vi "Write bestY.vi"(8 "error in (no error)":errorcluster, 10 "bestY":dbl, 11 "Utilities in":refnum<class "Utilities.lvclass">) -> (0 "error out":errorcluster, 3 "Utilities out":refnum<class "Utilities.lvclass">)   [LabVIEW 2023, in "Utilities.lvclass"]
uses:
  Utilities.lvclass
  Utilities.lvclass/Utilities.ctl
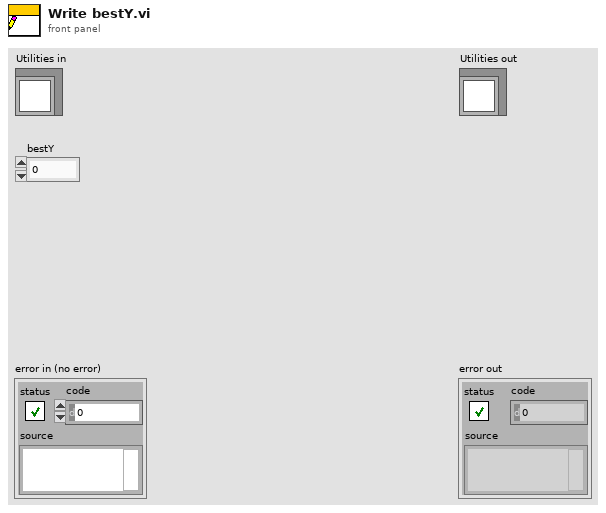
[diagram p1: front panel]
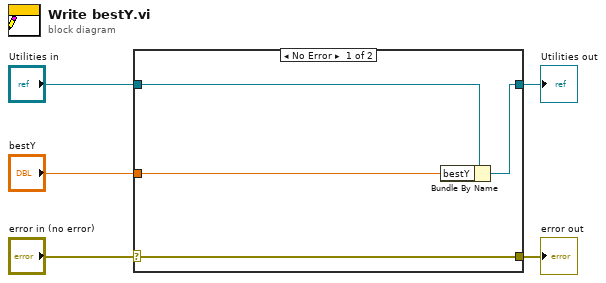
[diagram p0: block diagram]
diagram:
  n1 = case shown="No Error" "error in (no error)" {
    selector: "error in (no error)" -> [w9 w10]
    tunnel: [w9 w10] -> w4
    tunnel: [w7 w11] -> w2
    tunnel: "Utilities in" -> [w8 w11]
    tunnel: "bestY" -> [w6 _]
    frame No Error {
      n2 = Bundle By Name(cluster=w8, "bestY"=w6) -> (w7:refnum<class "Utilities.lvclass">)
    }
    frame Error {
    }
  }
  "error out" <- w4
  "Utilities out" <- w2
